vi "Main.vi"(7 "sweep rate, /min":dbl=0.2, 8 "sweep to:":dbl=-0.5, 9 "sweep":T3(radio)=enum."time_sweep") -> ()   [LabVIEW 2017] (continued)
                    n1197 = Build Array (concatenate)(w1474, w1473) -> (w1472:string[])
                    n1198 = Concatenate Strings(w1477, w1473, "\t") -> (w1476:string)
                  }
                }
                n1199 = property on="Figure_axis" class="Arr (strict)"("Value"=w1465) -> ()  [unwired: 2 in, 2 out]
                n1200 = property on="data_caption" class="Str"("Value"=w1467) -> ()  [unwired: 2 in, 2 out]
              }
              frame #14 {
                # "2182A 1 channel 1 measure (2182A_1_ch1)"
                n1201 = local read "2182A 1 ch1"() -> (w1484:bool)
                n1202 = property on="Figure_axis" class="Arr (strict)"() -> ("Value"=w1481:string[])  [unwired: 2 in, 2 out]
                n1203 = property on="data_caption" class="Str"() -> ("Value"=w1483:string)  [unwired: 2 in, 2 out]
                n1204 = case shown="False" w1484 {
                  tunnel: w1483 -> [w1486 w1492]
                  tunnel: [w1486 w1491] -> w1482
                  tunnel: w1481 -> [w1485 w1489]
                  tunnel: [w1485 w1487] -> w1480
                  frame False {
                    # "not measure 2182A 1 channel 1 (2182A_1_ch1)"
                  }
                  frame True {
                    w1488 = "2182A_1_ch1"
                    # "measure 2182A 1 channel 1 (2182A_1_ch1)"
                    n1205 = local read "2182A 1 addr"() -> (w1493:u8)
                    n1206 = Number To Decimal String(number=w1493) -> (decimal integer string=w1494:string)  [unwired: 1 in]
                    n1207 = GPIB Clear(3:w1494) -> ()  [unwired: 1 in, 2 out]
                    n1208 = Build Array (concatenate)(w1489, w1488) -> (w1487:string[])
                    n1209 = Concatenate Strings(w1492, w1488, "\t") -> (w1491:string)
                  }
                }
                n1210 = property on="Figure_axis" class="Arr (strict)"("Value"=w1480) -> ()  [unwired: 2 in, 2 out]
                n1211 = property on="data_caption" class="Str"("Value"=w1482) -> ()  [unwired: 2 in, 2 out]
              }
              frame #15 {
                # "2182A 1 channel 2 measure (2182A_1_ch2)"
                n1212 = local read "2182A 1 ch2"() -> (w1499:bool)
                n1213 = property on="Figure_axis" class="Arr (strict)"() -> ("Value"=w1496:string[])  [unwired: 2 in, 2 out]
                n1214 = property on="data_caption" class="Str"() -> ("Value"=w1498:string)  [unwired: 2 in, 2 out]
                n1215 = case shown="True" w1499 {
                  tunnel: w1498 -> [w1501 w1507]
                  tunnel: [w1501 w1506] -> w1497
                  tunnel: w1496 -> [w1500 w1504]
                  tunnel: [w1500 w1502] -> w1495
                  frame False {
                    # "not measure 2182A 1 channel 2 (2182A_1_ch2)"
                  }
                  frame True {
                    w1503 = "2182A_1_ch2"
                    # "measure 2182A 1 channel 2 (2182A_1_ch2)"
                    n1216 = local read "2182A 1 addr"() -> (w1508:u8)
                    n1217 = Number To Decimal String(number=w1508) -> (decimal integer string=w1509:string)  [unwired: 1 in]
                    n1218 = GPIB Clear(3:w1509) -> ()  [unwired: 1 in, 2 out]
                    n1219 = Build Array (concatenate)(w1504, w1503) -> (w1502:string[])
                    n1220 = Concatenate Strings(w1507, w1503, "\t") -> (w1506:string)
                  }
                }
                n1221 = property on="Figure_axis" class="Arr (strict)"("Value"=w1495) -> ()  [unwired: 2 in, 2 out]
                n1222 = property on="data_caption" class="Str"("Value"=w1497) -> ()  [unwired: 2 in, 2 out]
              }
              frame #16 {
                # "2182A 2 channel 1 measure (2182A_2_ch1)"
                n1223 = local read "2182A 2 ch1"() -> (w1514:bool)
                n1224 = property on="Figure_axis" class="Arr (strict)"() -> ("Value"=w1511:string[])  [unwired: 2 in, 2 out]
                n1225 = property on="data_caption" class="Str"() -> ("Value"=w1513:string)  [unwired: 2 in, 2 out]
                n1226 = case shown="True" w1514 {
                  tunnel: w1513 -> [w1516 w1522]
                  tunnel: [w1516 w1521] -> w1512
                  tunnel: w1511 -> [w1515 w1519]
                  tunnel: [w1515 w1517] -> w1510
                  frame False {
                    # "not measure 2182A 2 channel 1 (2182A_2_ch1)"
                  }
                  frame True {
                    w1518 = "2182A_2_ch1"
                    # "measure 2182A 2 channel 1 (2182A_2_ch1)"
                    n1227 = local read "2182A 2 addr"() -> (w1523:u8)
                    n1228 = Number To Decimal String(number=w1523) -> (decimal integer string=w1524:string)  [unwired: 1 in]
                    n1229 = GPIB Clear(3:w1524) -> ()  [unwired: 1 in, 2 out]
                    n1230 = Build Array (concatenate)(w1519, w1518) -> (w1517:string[])
                    n1231 = Concatenate Strings(w1522, w1518, "\t") -> (w1521:string)
                  }
                }
                n1232 = property on="Figure_axis" class="Arr (strict)"("Value"=w1510) -> ()  [unwired: 2 in, 2 out]
                n1233 = property on="data_caption" class="Str"("Value"=w1512) -> ()  [unwired: 2 in, 2 out]
              }
              frame #17 {
                # "2182A 2 channel 2 measure (2182A_2_ch2)"
                n1234 = local read "2182A 2 ch2"() -> (w1529:bool)
                n1235 = property on="Figure_axis" class="Arr (strict)"() -> ("Value"=w1526:string[])  [unwired: 2 in, 2 out]
                n1236 = property on="data_caption" class="Str"() -> ("Value"=w1528:string)  [unwired: 2 in, 2 out]
                n1237 = case shown="True" w1529 {
                  tunnel: w1528 -> [w1531 w1537]
                  tunnel: [w1531 w1536] -> w1527
                  tunnel: w1526 -> [w1530 w1534]
                  tunnel: [w1530 w1532] -> w1525
                  frame False {
                    # "not measure 2182A 2 channel 2 (2182A_2_ch2)"
                  }
                  frame True {
                    w1533 = "2182A_2_ch2"
                    # "measure 2182A 2 channel 2 (2182A_2_ch2)"
                    n1238 = local read "2182A 2 addr"() -> (w1538:u8)
                    n1239 = Number To Decimal String(number=w1538) -> (decimal integer string=w1539:string)  [unwired: 1 in]
                    n1240 = GPIB Clear(3:w1539) -> ()  [unwired: 1 in, 2 out]
                    n1241 = Build Array (concatenate)(w1534, w1533) -> (w1532:string[])
                    n1242 = Concatenate Strings(w1537, w1533, "\t") -> (w1536:string)
                  }
                }
                n1243 = property on="Figure_axis" class="Arr (strict)"("Value"=w1525) -> ()  [unwired: 2 in, 2 out]
                n1244 = property on="data_caption" class="Str"("Value"=w1527) -> ()  [unwired: 2 in, 2 out]
              }
              frame #18 {
                # "2182A 3 channel 1 measure (2182A_3_ch1)"
                n1245 = local read "2182A 3 ch1"() -> (w1544:bool)
                n1246 = property on="Figure_axis" class="Arr (strict)"() -> ("Value"=w1541:string[])  [unwired: 2 in, 2 out]
                n1247 = property on="data_caption" class="Str"() -> ("Value"=w1543:string)  [unwired: 2 in, 2 out]
                n1248 = case shown="True" w1544 {
                  tunnel: w1543 -> [w1546 w1552]
                  tunnel: [w1546 w1551] -> w1542
                  tunnel: w1541 -> [w1545 w1549]
                  tunnel: [w1545 w1547] -> w1540
                  frame False {
                    # "not measure 2182A 3 channel 1 (2182A_3_ch1)"
                  }
                  frame True {
                    w1548 = "2182A_3_ch1"
                    # "measure 2182A 3 channel 1 (2182A_3_ch1)"
                    n1249 = local read "2182A 3 addr"() -> (w1553:u8)
                    n1250 = Number To Decimal String(number=w1553) -> (decimal integer string=w1554:string)  [unwired: 1 in]
                    n1251 = GPIB Clear(3:w1554) -> ()  [unwired: 1 in, 2 out]
                    n1252 = Build Array (concatenate)(w1549, w1548) -> (w1547:string[])
                    n1253 = Concatenate Strings(w1552, w1548, "\t") -> (w1551:string)
                  }
                }
                n1254 = property on="Figure_axis" class="Arr (strict)"("Value"=w1540) -> ()  [unwired: 2 in, 2 out]
                n1255 = property on="data_caption" class="Str"("Value"=w1542) -> ()  [unwired: 2 in, 2 out]
              }
              frame #19 {
                # "2182A 3 channel 2 measure (2182A_3_ch2)"
                n1256 = local read "2182A 3 ch2"() -> (w1559:bool)
                n1257 = property on="Figure_axis" class="Arr (strict)"() -> ("Value"=w1556:string[])  [unwired: 2 in, 2 out]
                n1258 = property on="data_caption" class="Str"() -> ("Value"=w1558:string)  [unwired: 2 in, 2 out]
                n1259 = case shown="False" w1559 {
                  tunnel: w1558 -> [w1561 w1567]
                  tunnel: [w1561 w1566] -> w1557
                  tunnel: w1556 -> [w1560 w1564]
                  tunnel: [w1560 w1562] -> w1555
                  frame False {
                    # "not measure 2182A 3 channel 2 (2182A_3_ch2)"
                  }
                  frame True {
                    w1563 = "2182A_3_ch2"
                    # "measure 2182A 3 channel 2 (2182A_3_ch2)"
                    n1260 = local read "2182A 3 addr"() -> (w1568:u8)
                    n1261 = Number To Decimal String(number=w1568) -> (decimal integer string=w1569:string)  [unwired: 1 in]
                    n1262 = GPIB Clear(3:w1569) -> ()  [unwired: 1 in, 2 out]
                    n1263 = Build Array (concatenate)(w1564, w1563) -> (w1562:string[])
                    n1264 = Concatenate Strings(w1567, w1563, "\t") -> (w1566:string)
                  }
                }
                n1265 = property on="Figure_axis" class="Arr (strict)"("Value"=w1555) -> ()  [unwired: 2 in, 2 out]
                n1266 = property on="data_caption" class="Str"("Value"=w1557) -> ()  [unwired: 2 in, 2 out]
              }
              frame #20 {
                # "2182A 4 channel 1 measure (2182A_4_ch1)"
                n1267 = local read "2182A 4 ch1"() -> (w1574:bool)
                n1268 = property on="Figure_axis" class="Arr (strict)"() -> ("Value"=w1571:string[])  [unwired: 2 in, 2 out]
                n1269 = property on="data_caption" class="Str"() -> ("Value"=w1573:string)  [unwired: 2 in, 2 out]
                n1270 = case shown="True" w1574 {
                  tunnel: w1573 -> [w1576 w1582]
                  tunnel: [w1576 w1581] -> w1572
                  tunnel: w1571 -> [w1575 w1579]
                  tunnel: [w1575 w1577] -> w1570
                  frame False {
                    # "not measure 2182A 4 channel 1 (2182A_4_ch1)"
                  }
                  frame True {
                    w1578 = "2182A_4_ch1"
                    # "measure 2182A 4 channel 1 (2182A_4_ch1)"
                    n1271 = local read "2182A 4 addr"() -> (w1583:u8)
                    n1272 = Number To Decimal String(number=w1583) -> (decimal integer string=w1584:string)  [unwired: 1 in]
                    n1273 = GPIB Clear(3:w1584) -> ()  [unwired: 1 in, 2 out]
                    n1274 = Build Array (concatenate)(w1579, w1578) -> (w1577:string[])
                    n1275 = Concatenate Strings(w1582, w1578, "\t") -> (w1581:string)
                  }
                }
                n1276 = property on="Figure_axis" class="Arr (strict)"("Value"=w1570) -> ()  [unwired: 2 in, 2 out]
                n1277 = property on="data_caption" class="Str"("Value"=w1572) -> ()  [unwired: 2 in, 2 out]
              }
              frame #21 {
                # "2182A 4 channel 2 measure (2182A_4_ch2)"
                n1278 = local read "2182A 4 ch2"() -> (w1589:bool)
                n1279 = property on="Figure_axis" class="Arr (strict)"() -> ("Value"=w1586:string[])  [unwired: 2 in, 2 out]
                n1280 = property on="data_caption" class="Str"() -> ("Value"=w1588:string)  [unwired: 2 in, 2 out]
                n1281 = case shown="True" w1589 {
                  tunnel: w1588 -> [w1591 w1597]
                  tunnel: [w1591 w1596] -> w1587
                  tunnel: w1586 -> [w1590 w1594]
                  tunnel: [w1590 w1592] -> w1585
                  frame False {
                    # "not measure 2182A 4 channel 2 (2182A_4_ch2)"
                  }
                  frame True {
                    w1593 = "2182A_4_ch2"
                    # "measure 2182A 4 channel 2 (2182A_4_ch2)"
                    n1282 = local read "2182A 4 addr"() -> (w1598:u8)
                    n1283 = Number To Decimal String(number=w1598) -> (decimal integer string=w1599:string)  [unwired: 1 in]
                    n1284 = GPIB Clear(3:w1599) -> ()  [unwired: 1 in, 2 out]
                    n1285 = Build Array (concatenate)(w1594, w1593) -> (w1592:string[])
                    n1286 = Concatenate Strings(w1597, w1593, "\t") -> (w1596:string)
                  }
                }
                n1287 = property on="Figure_axis" class="Arr (strict)"("Value"=w1585) -> ()  [unwired: 2 in, 2 out]
                n1288 = property on="data_caption" class="Str"("Value"=w1587) -> ()  [unwired: 2 in, 2 out]
              }
              frame #22 {
                # "2636A smua measure voltage (2636A_smua_v)"
                n1289 = local read "2636A smua meas v"() -> (w1604:bool)
                n1290 = property on="Figure_axis" class="Arr (strict)"() -> ("Value"=w1601:string[])  [unwired: 2 in, 2 out]
                n1291 = property on="data_caption" class="Str"() -> ("Value"=w1603:string)  [unwired: 2 in, 2 out]
                n1292 = case shown="True" w1604 {
                  tunnel: w1603 -> [w1606 w1617]
                  tunnel: [w1606 w1616] -> w1602
                  tunnel: w1601 -> [w1605 w1614]
                  tunnel: [w1605 w1612] -> w1600
                  frame False {
                    # "not measure voltage on 2636A smua (2636A_smua_v)"
                  }
                  frame True {
                    w1613 = "2636A_smua_v"
                    # "measure voltage on 2636A smua (2636A_smua_v)"
                    n1293 = local read "2336A addr"() -> (w1608:refnum<visa-resource-name>)
                    n1294 = VISA Open(VISA resource name=w1608) -> (VISA resource name=w1607:refnum<visa-resource-name>, error out=w1609:errorcluster)  [unwired: 4 in]
                    n1295 = VISA Clear(VISA resource name=w1607, error in (no error)=w1609) -> (VISA resource name out=w1611:refnum<visa-resource-name>)  [unwired: 1 out]
                    n1296 = property class="Instr"(reference=w1611, "General Settings:Timeout Value"=u32 10000) -> ()  [unwired: 1 in, 2 out]
                    n1297 = Build Array (concatenate)(w1614, w1613) -> (w1612:string[])
                    n1298 = Concatenate Strings(w1617, w1613, "\t") -> (w1616:string)
                  }
                }
                n1299 = property on="Figure_axis" class="Arr (strict)"("Value"=w1600) -> ()  [unwired: 2 in, 2 out]
                n1300 = property on="data_caption" class="Str"("Value"=w1602) -> ()  [unwired: 2 in, 2 out]
              }
              frame #23 {
                # "2636A smua measure current (2636A_smua_i)"
                n1301 = local read "2636A smua meas i"() -> (w1622:bool)
                n1302 = property on="Figure_axis" class="Arr (strict)"() -> ("Value"=w1619:string[])  [unwired: 2 in, 2 out]
                n1303 = property on="data_caption" class="Str"() -> ("Value"=w1621:string)  [unwired: 2 in, 2 out]
                n1304 = case shown="True" w1622 {
                  tunnel: w1621 -> [w1624 w1635]
                  tunnel: [w1624 w1634] -> w1620
                  tunnel: w1619 -> [w1623 w1632]
                  tunnel: [w1623 w1630] -> w1618
                  frame False {
                    # "not measure current on 2636A smua (2636A_smua_i)"
                  }
                  frame True {
                    w1631 = "2636A_smua_i"
                    # "measure current on 2636A smua (2636A_smua_i)"
                    n1305 = local read "2336A addr"() -> (w1627:refnum<visa-resource-name>)
                    n1306 = VISA Open(VISA resource name=w1627) -> (VISA resource name=w1626:refnum<visa-resource-name>, error out=w1625:errorcluster)  [unwired: 4 in]
                    n1307 = VISA Clear(VISA resource name=w1626, error in (no error)=w1625) -> (VISA resource name out=w1628:refnum<visa-resource-name>)  [unwired: 1 out]
                    n1308 = Build Array (concatenate)(w1632, w1631) -> (w1630:string[])
                    n1309 = property class="Instr"(reference=w1628, "General Settings:Timeout Value"=u32 10000) -> ()  [unwired: 1 in, 2 out]
                    n1310 = Concatenate Strings(w1635, w1631, "\t") -> (w1634:string)
                  }
                }
                n1311 = property on="Figure_axis" class="Arr (strict)"("Value"=w1618) -> ()  [unwired: 2 in, 2 out]
                n1312 = property on="data_caption" class="Str"("Value"=w1620) -> ()  [unwired: 2 in, 2 out]
              }
              frame #24 {
                # "2636A smub measure voltage (2636A_smub_v)"
                n1313 = local read "2636A smub meas v"() -> (w1640:bool)
                n1314 = property on="Figure_axis" class="Arr (strict)"() -> ("Value"=w1637:string[])  [unwired: 2 in, 2 out]
                n1315 = property on="data_caption" class="Str"() -> ("Value"=w1639:string)  [unwired: 2 in, 2 out]
                n1316 = case shown="True" w1640 {
                  tunnel: w1639 -> [w1642 w1653]
                  tunnel: [w1642 w1652] -> w1638
                  tunnel: w1637 -> [w1641 w1650]
                  tunnel: [w1641 w1648] -> w1636
                  frame False {
                    # "not measure voltage on 2636A smub (2636A_smub_v)"
                  }
                  frame True {
                    w1649 = "2636A_smub_v"
                    # "measure voltage on 2636A smub (2636A_smub_v)"
                    n1317 = local read "2336A addr"() -> (w1644:refnum<visa-resource-name>)
                    n1318 = VISA Open(VISA resource name=w1644) -> (VISA resource name=w1643:refnum<visa-resource-name>, error out=w1645:errorcluster)  [unwired: 4 in]
                    n1319 = VISA Clear(VISA resource name=w1643, error in (no error)=w1645) -> (VISA resource name out=w1646:refnum<visa-resource-name>)  [unwired: 1 out]
                    n1320 = Build Array (concatenate)(w1650, w1649) -> (w1648:string[])
                    n1321 = property class="Instr"(reference=w1646, "General Settings:Timeout Value"=u32 10000) -> ()  [unwired: 1 in, 2 out]
                    n1322 = Concatenate Strings(w1653, w1649, "\t") -> (w1652:string)
                  }
                }
                n1323 = property on="Figure_axis" class="Arr (strict)"("Value"=w1636) -> ()  [unwired: 2 in, 2 out]
                n1324 = property on="data_caption" class="Str"("Value"=w1638) -> ()  [unwired: 2 in, 2 out]
              }
              frame #25 {
                # "2636A smub measure current (2636A_smub_i)"
                n1325 = local read "2636A smub meas i"() -> (w1658:bool)
                n1326 = property on="Figure_axis" class="Arr (strict)"() -> ("Value"=w1655:string[])  [unwired: 2 in, 2 out]
                n1327 = property on="data_caption" class="Str"() -> ("Value"=w1657:string)  [unwired: 2 in, 2 out]
                n1328 = case shown="True" w1658 {
                  tunnel: w1657 -> [w1660 w1671]
                  tunnel: [w1660 w1670] -> w1656
                  tunnel: w1655 -> [w1659 w1668]
                  tunnel: [w1659 w1666] -> w1654
                  frame False {
                    # "not measure current on 2636A smub (2636A_smub_i)"
                  }
                  frame True {
                    w1667 = "2636A_smub_i"
                    # "measure current on 2636A smub (2636A_smub_i)"
                    n1329 = local read "2336A addr"() -> (w1661:refnum<visa-resource-name>)
                    n1330 = VISA Open(VISA resource name=w1661) -> (VISA resource name=w1662:refnum<visa-resource-name>, error out=w1663:errorcluster)  [unwired: 4 in]
                    n1331 = VISA Clear(VISA resource name=w1662, error in (no error)=w1663) -> (VISA resource name out=w1664:refnum<visa-resource-name>)  [unwired: 1 out]
                    n1332 = Build Array (concatenate)(w1668, w1667) -> (w1666:string[])
                    n1333 = property class="Instr"(reference=w1664, "General Settings:Timeout Value"=u32 10000) -> ()  [unwired: 1 in, 2 out]
                    n1334 = Concatenate Strings(w1671, w1667, "\t") -> (w1670:string)
                  }
                }
                n1335 = property on="Figure_axis" class="Arr (strict)"("Value"=w1654) -> ()  [unwired: 2 in, 2 out]
                n1336 = property on="data_caption" class="Str"("Value"=w1656) -> ()  [unwired: 2 in, 2 out]
              }
              frame #26 {
                # "measure time"
                n1337 = local read "measure time"() -> (w1676:bool)
                n1338 = property on="Figure_axis" class="Arr (strict)"() -> ("Value"=w1673:string[])  [unwired: 2 in, 2 out]
                n1339 = property on="data_caption" class="Str"() -> ("Value"=w1675:string)  [unwired: 2 in, 2 out]
                n1340 = case shown="True" w1676 {
                  tunnel: w1675 -> [w1678 w1684]
                  tunnel: [w1678 w1683] -> w1674
                  tunnel: w1673 -> [w1677 w1681]
                  tunnel: [w1677 w1679] -> w1672
                  frame False {
                    # "not measuring time"
                  }
                  frame True {
                    w1680 = "time"
                    # "measuring time"
                    n1341 = Build Array (concatenate)(w1681, w1680) -> (w1679:string[])
                    n1342 = Concatenate Strings(w1684, w1680, "\t") -> (w1683:string)
                  }
                }
                n1343 = property on="Figure_axis" class="Arr (strict)"("Value"=w1672) -> ()  [unwired: 2 in, 2 out]
                n1344 = property on="data_caption" class="Str"("Value"=w1674) -> ()  [unwired: 2 in, 2 out]
              }
              frame #27 {
                # "Measure magnetic field on IPS120-0"
                n1345 = local read "iPS_MagnetField"() -> (w1689:bool)
                n1346 = property on="Figure_axis" class="Arr (strict)"() -> ("Value"=w1686:string[])  [unwired: 2 in, 2 out]
                n1347 = property on="data_caption" class="Str"() -> ("Value"=w1688:string)  [unwired: 2 in, 2 out]
                n1348 = case shown="True" w1689 {
                  tunnel: w1688 -> [w1691 w1699]
                  tunnel: [w1691 w1698] -> w1687
                  tunnel: w1686 -> [w1690 w1696]
                  tunnel: [w1690 w1694] -> w1685
                  frame False {
                    # "do not Measure magnetic field on IPS120-0"
                  }
                  frame True {
                    w1695 = "iPS_MagntField"
                    n1349 = local read "IPS120-0 addr_sweep"() -> (w1693:u8)
                    n1350 = Number To Decimal String(number=w1693) -> (decimal integer string=w1692:string)  [unwired: 1 in]
                    n1351 = GPIB Clear(3:w1692) -> ()  [unwired: 1 in, 2 out]
                    n1352 = Build Array (concatenate)(w1696, w1695) -> (w1694:string[])
                    n1353 = Concatenate Strings(w1699, w1695, "\t") -> (w1698:string)
                  }
                }
                n1354 = property on="Figure_axis" class="Arr (strict)"("Value"=w1685) -> ()  [unwired: 2 in, 2 out]
                n1355 = property on="data_caption" class="Str"("Value"=w1687) -> ()  [unwired: 2 in, 2 out]
              }
              frame #28 {
                # "iTC sample Temp"
                n1356 = property on="iTC_Sample_T" class="Bool (strict)"() -> ("Value"=w1700:bool)  [unwired: 2 in, 2 out]
                n1357 = property on="Figure_axis" class="Arr (strict)"() -> ("Value"=w1702:string[])  [unwired: 2 in, 2 out]
                n1358 = property on="data_caption" class="Str"() -> ("Value"=w1704:string)  [unwired: 2 in, 2 out]
                n1359 = case shown="True" w1700 {
                  tunnel: w1704 -> [w1706 w1714]
                  tunnel: [w1706 w1713] -> w1703
                  tunnel: w1702 -> [w1705 w1711]
                  tunnel: [w1705 w1709] -> w1701
                  frame False {
                    # "not measure 2461 voltage (2461_meas_v)"
                  }
                  frame True {
                    w1710 = "iTC_Sample_T"
                    n1360 = local read "ITC503S addr_step"() -> (w1708:u8)
                    n1361 = Number To Decimal String(number=w1708) -> (decimal integer string=w1707:string)  [unwired: 1 in]
                    n1362 = GPIB Clear(3:w1707) -> ()  [unwired: 1 in, 2 out]
                    n1363 = Build Array (concatenate)(w1711, w1710) -> (w1709:string[])
                    n1364 = Concatenate Strings(w1714, w1710, "\t") -> (w1713:string)
                  }
                }
                n1365 = property on="Figure_axis" class="Arr (strict)"("Value"=w1701) -> ()  [unwired: 2 in, 2 out]
                n1366 = property on="data_caption" class="Str"("Value"=w1703) -> ()  [unwired: 2 in, 2 out]
              }
              frame #29 {
                # "iTC CH_A Temp"
                n1367 = property on="CH_A" class="Bool (strict)"() -> ("Value"=w1715:bool)  [unwired: 2 in, 2 out]
                n1368 = property on="Figure_axis" class="Arr (strict)"() -> ("Value"=w1717:string[])  [unwired: 2 in, 2 out]
                n1369 = property on="data_caption" class="Str"() -> ("Value"=w1719:string)  [unwired: 2 in, 2 out]
                n1370 = case shown="True" w1715 {
                  tunnel: w1719 -> [w1721 w1727]
                  tunnel: [w1721 w1726] -> w1718
                  tunnel: w1717 -> [w1720 w1724]
                  tunnel: [w1720 w1722] -> w1716
                  frame False {
                    # "not measure 2461 voltage (2461_meas_v)"
                  }
                  frame True {
                    w1723 = "iTC_CH_A"
                    n1371 = Build Array (concatenate)(w1724, w1723) -> (w1722:string[])
                    n1372 = Concatenate Strings(w1727, w1723, "\t") -> (w1726:string)
                  }
                }
                n1373 = property on="Figure_axis" class="Arr (strict)"("Value"=w1716) -> ()  [unwired: 2 in, 2 out]
                n1374 = property on="data_caption" class="Str"("Value"=w1718) -> ()  [unwired: 2 in, 2 out]
              }
              frame #30 {
                # "iTC sample Temp"
                n1375 = property on="CH_B" class="Bool (strict)"() -> ("Value"=w1728:bool)  [unwired: 2 in, 2 out]
                n1376 = property on="Figure_axis" class="Arr (strict)"() -> ("Value"=w1730:string[])  [unwired: 2 in, 2 out]
                n1377 = property on="data_caption" class="Str"() -> ("Value"=w1732:string)  [unwired: 2 in, 2 out]
                n1378 = case shown="True" w1728 {
                  tunnel: w1732 -> [w1734 w1740]
                  tunnel: [w1734 w1739] -> w1731
                  tunnel: w1730 -> [w1733 w1737]
                  tunnel: [w1733 w1735] -> w1729
                  frame False {
                    # "not measure 2461 voltage (2461_meas_v)"
                  }
                  frame True {
                    w1736 = "iTC_CH_B"
                    n1379 = Build Array (concatenate)(w1737, w1736) -> (w1735:string[])
                    n1380 = Concatenate Strings(w1740, w1736, "\t") -> (w1739:string)
                  }
                }
                n1381 = property on="Figure_axis" class="Arr (strict)"("Value"=w1729) -> ()  [unwired: 2 in, 2 out]
                n1382 = property on="data_caption" class="Str"("Value"=w1731) -> ()  [unwired: 2 in, 2 out]
              }
              frame #31 {
                # "iTC sample Temp"
                n1383 = property on="Linetrace or Mapping?" class="Bool (strict)"() -> ("Value"=w1741:bool)  [unwired: 2 in, 2 out]
                n1384 = property on="Figure_axis" class="Arr (strict)"() -> ("Value"=w1743:string[])  [unwired: 2 in, 2 out]
                n1385 = property on="data_caption" class="Str"() -> ("Value"=w1745:string)  [unwired: 2 in, 2 out]
                n1386 = case shown="True" w1741 {
                  tunnel: w1745 -> [w1747 w1753]
                  tunnel: [w1747 w1752] -> w1744
                  tunnel: w1743 -> [w1746 w1750]
                  tunnel: [w1746 w1748] -> w1742
                  frame False {
                    # "not measure 2461 voltage (2461_meas_v)"
                  }
                  frame True {
                    w1749 = "Step_Value"
                    n1387 = Build Array (concatenate)(w1750, w1749) -> (w1748:string[])
                    n1388 = Concatenate Strings(w1753, w1749, "\t") -> (w1752:string)
                  }
                }
                n1389 = property on="Figure_axis" class="Arr (strict)"("Value"=w1742) -> ()  [unwired: 2 in, 2 out]
                n1390 = property on="data_caption" class="Str"("Value"=w1744) -> ()  [unwired: 2 in, 2 out]
              }
            }
          }
          frame #2 {
            # "1 = 2400 1\n2 = 2400 2\n3 = 2400 3\n4 = 2636a smua\n5 = 2636a smub\n6 = do not sweep, just time\n7 = Teslatron_iPS_Field\n8 = Teslatron_iTC_Sample T"
            n1391 = property on="sweep" class="RadioBtnsControl (strict)"() -> ("Value"=w1754:T3)  [unwired: 2 in, 2 out]
            n1392 = case "reads current value from instrument which will be sweeping" shown="\"2636a_smub\"" w1754 {
              tunnel: [w1756 w1766 w1775 w1784 w1788 0.0 ("Measuremet") w1794 w1795] -> w1755
              frame "2400_1", Default {
                # "reads the voltage on 2400 1"
                n1393 = local read "2400 1 addr"() -> (w1760:u8)
                n1394 = Number To Decimal String(number=w1760) -> (decimal integer string=w1761:string)  [unwired: 1 in]
                n1395 = GPIB Write(0:w1761, 1:":READ?") -> (6:w1757:errorcluster)  [unwired: 3 in, 1 out]
                n1396 = GPIB Read(0:w1761, 1:3200, 3:w1757) -> (5:w1763:string)  [unwired: 2 in, 2 out]
                n1397 = String Subset(string=w1763, length (rest)=13) -> (substring=w1764:string)  [unwired: 1 in]
                n1398 = Fract/Exp String To Number(string=w1764) -> (number=w1756:dbl)  [unwired: 3 in, 1 out]
              }
              frame "2400_2" {
                # "reads the current on 2400 2"
                n1399 = local read "2400 2 addr"() -> (w1770:u8)
                n1400 = Number To Decimal String(number=w1770) -> (decimal integer string=w1771:string)  [unwired: 1 in]
                n1401 = GPIB Write(0:w1771, 1:":READ?") -> (6:w1767:errorcluster)  [unwired: 3 in, 1 out]
                n1402 = GPIB Read(0:w1771, 1:3200, 3:w1767) -> (5:w1773:string)  [unwired: 2 in, 2 out]
                n1403 = String Subset(string=w1773, offset (0)=14, length (rest)=13) -> (substring=w1774:string)
                n1404 = Fract/Exp String To Number(string=w1774) -> (number=w1766:dbl)  [unwired: 3 in, 1 out]
              }
              frame "2400_3" {
                # "reads the voltage on 2400 3"
                n1405 = local read "2400 3 addr"() -> (w1779:u8)
                n1406 = Number To Decimal String(number=w1779) -> (decimal integer string=w1780:string)  [unwired: 1 in]
                n1407 = GPIB Write(0:w1780, 1:":READ?") -> (6:w1776:errorcluster)  [unwired: 3 in, 1 out]
                n1408 = GPIB Read(0:w1780, 1:3200, 3:w1776) -> (5:w1782:string)  [unwired: 2 in, 2 out]
                n1409 = String Subset(string=w1782, length (rest)=13) -> (substring=w1783:string)  [unwired: 1 in]
                n1410 = Fract/Exp String To Number(string=w1783) -> (number=w1775:dbl)  [unwired: 3 in, 1 out]
              }
              frame "2636a_smua" {
                # "reads the voltage on 2636a smua"
                n1411 = local read "2336A addr"() -> (w1787:refnum<visa-resource-name>)
                n1412 = call "SinglePointMeasurement.vi"("Measure"=Measure."Voltage", "Channel"=Channel."a", "VISA resource name 2"=w1787) -> ("Measuremet"=w1784:dbl)  [unwired: 3 in, 4 out]
              }
              frame "2636a_smub" {
                # "reads the voltage on 2636a smub"
                n1413 = local read "2336A addr"() -> (w1791:refnum<visa-resource-name>)
                n1414 = call "SinglePointMeasurement.vi"("Measure"=Measure."Voltage", "Channel"=Channel."b", "VISA resource name 2"=w1791) -> ("Measuremet"=w1788:dbl)  [unwired: 3 in, 4 out]
              }
              frame "time_sweep" {
              }
              frame "iPS" {
                # "Measure magnetic field on IPS120-0"
                n1415 = call "iPSread.vi"("iPSreadCtrl"=iPSreadCtrl."OutputField") -> ("number"=w1794:dbl)  [unwired: 7 in, 3 out]
              }
              frame "iTC" {
                n1416 = call "iTCread.vi"("iTCreadCtrl"=iTCreadCtrl."Sample Temp") -> ("number"=w1795:dbl)  [unwired: 6 in, 3 out]
              }
            }
          }
          frame #3 {
            n1417 = property on="Linetrace or Mapping?" class="Bool (strict)"() -> ("Value"=w1797:bool)  [unwired: 2 in, 2 out]
            n1418 = case shown="True" w1797 {
              frame False {
                # "Reserve a name for new linetrace data file:"
                n1419 = property on="Data Folder" class="Path"() -> ("Value"=w1805:path)  [unwired: 2 in, 2 out]
                n1420 = call "AutoNamerDatExtraArtem.vi"("SweepType"="linetraces", "Custom User Path"=w1805) -> ("String"=w1803:string, "Path"=w1804:path)  [unwired: 2 in]
                n1421 = Path To String(path=w1804) -> (string=w1802:string)
                n1422 = Concatenate Strings(w1802, "\\", w1803) -> (w1801:string)
                n1423 = String To Path(string=w1801) -> (path=w1800:path)
                n1424 = local write "Data file:"(w1800) -> ()
              }
              frame True {
                n1425 = property on="Sweep Direction" class="Str"() -> ("Value"=w1806:string)  [unwired: 2 in, 2 out]
                n1426 = case shown="\"Sweep Down\"" w1806 {
                  frame "Sweep Up" {
                    n1427 = property on="UpNameString" class="Str"() -> ("Value"=w1808:string)  [unwired: 2 in, 2 out]
                    n1428 = String To Path(string=w1808) -> (path=w1807:path)
                    n1429 = local write "Data file:"(w1807) -> ()
                  }
                  frame "Sweep Down" {
                    n1430 = property on="DownNameString" class="Str"() -> ("Value"=w1809:string)  [unwired: 2 in, 2 out]
                    n1431 = String To Path(string=w1809) -> (path=w1810:path)
                    n1432 = local write "Data file:"(w1810) -> ()
                  }
                  frame "Ramp Down", Default {
                  }
                }
              }
            }
          }
          frame #4 {
            # "add \"formula\" string to the axis rings"
            n1433 = property on="Figure_axis" class="Arr (strict)"() -> ("Value"=w1813:string[])  [unwired: 2 in, 2 out]
            n1434 = Build Array (concatenate)(w1813, "formula") -> (w1811:string[])
            n1435 = property on="Figure_axis" class="Arr (strict)"("Value"=w1811) -> ()  [unwired: 2 in, 2 out]
          }
          frame #5 {
            # "passes array to ring"
            n1436 = property on="Linetrace or Mapping?" class="Bool (strict)"() -> ("Value"=w1814:bool)  [unwired: 2 in, 2 out]
            n1437 = case shown="True" w1814 {
              frame False {
                # "records the fist line into the data file"
                n1438 = property on="data_caption" class="Str"() -> ("Value"=w1818:string)  [unwired: 2 in, 2 out]
                n1439 = local read "Data file:"() -> (w1819:path)
                n1440 = Concatenate Strings(w1818, "\r") -> (w1820:string)
                n1441 = Write to Text File(file (use dialog)=w1819, text=w1820) -> ()  [unwired: 2 in, 3 out]
              }
              frame True {
                # "records the fist line into the both upa nd down data file\nwhen table index=0"
                n1442 = property on="Table Index" class="DigNum (strict)"() -> ("Value"=w1822:dbl)  [unwired: 2 in, 2 out]
                n1443 = Equal To 0?(x=w1822) -> (x = 0?=w1821:bool)
                n1444 = case shown="True" w1821 {
                  frame False {
                  }
                  frame True {
                    n1445 = property on="data_caption" class="Str"() -> ("Value"=w1826:string)  [unwired: 2 in, 2 out]
                    n1446 = local read "Data file:"() -> (w1823:path)
                    n1447 = Concatenate Strings(w1826, "\r") -> (w1825:string)
                    n1448 = Write to Text File(file (use dialog)=w1823, text=w1825) -> ()  [unwired: 2 in, 3 out]
                  }
                }
              }
            }
            n1449 = property on="Figure_axis" class="Arr (strict)"() -> ("Value"=w1816:string[])  [unwired: 2 in, 2 out]
            n1450 = property on="Xaxis" class="Ring (strict)"("Strings []"=w1816) -> ()  [unwired: 2 in, 2 out]
            n1451 = property on="Stop Sweep" class="Bool"("DisabledEnum"=T5."Enabled" ("Disabled")) -> ()  [unwired: 2 in, 2 out]
            n1452 = property on="Yright" class="Ring (strict)"("Strings []"=w1816) -> ()  [unwired: 2 in, 2 out]
            n1453 = property on="Yaxis" class="Ring (strict)"("Strings []"=w1816) -> ()  [unwired: 2 in, 2 out]
          }
        }
        n1454 = while {
          shift-right: [w1877] -> _
          shift-left: w1212 -> [w1878]
          shift-right: [w1875] -> w1211
          shift-left: w1209 -> [w1874]
          tunnel: w1213 -> [w1872]
          stop <- w1864 stop-if-true
          # "initial value"
          # "Measure the selected channels"
          # "data array"
          # "this loop stops when target value is reached"
          # "error cluster to determine data flow"
          n1455 = stacked-sequence {
            tunnel: [_ _ w1894 _ _ _] -> w1865
            tunnel: [_ _ w1893 _ _ _] -> w1876
            tunnel: w1874 -> [_ _ w1888 _ _ _]
            tunnel: [w1884 _ _ _ _ _] -> w1873
            tunnel: w1872 -> [_ _ _ w1909 _ _]
            tunnel: [_ _ w1888 _ _ _] -> w1868
            tunnel: [_ _ _ _ _ w2369] -> w1863
            frame #0 {
              # "time is measured at the beginning\nand at the end of the cycle to\ncalculate delay time required to\nkeep set sweep rate"
              n1456 = flat-sequence {
                tunnel: [w1886] -> w1884
                frame #0 {
                  n1457 = property on="time delay, ms" class="DigNum (strict)"() -> ("Value"=w1885:dbl)  [unwired: 2 in, 2 out]
                  n1458 = Wait (ms)(milliseconds to wait=w1885) -> ()  [unwired: 1 out]
                }
                frame #1 {
                  n1459 = Tick Count (ms)() -> (millisecond timer value=w1886:u32)
                }
              }
            }
            frame #1 {
              w1887 = dbl[] []  # Empty array for data
              # "clear data array before each measurement cycle"
              n1460 = property on="data" class="Arr (strict)"("Value"=w1887) -> ()  [unwired: 2 in, 2 out]
            }
            frame #2 {
              # "add next sweep value to the data array"
              n1461 = property on="data" class="Arr (strict)"() -> ("Value"=w1892:dbl[])  [unwired: 2 in, 2 out]
              n1462 = case shown="False" FALSE {
                tunnel: [w1895 w1905] -> w1894
                tunnel: [w1896 w1904] -> w1893
                tunnel: w1888 -> [_ w1902]
                tunnel: [w1896 w1902] -> w1890
                frame True {
                  # "sweeping magnetic field of Hulk"
                  n1463 = stacked-sequence {
                    tunnel: [_ w1898 _] -> w1896
                    tunnel: [_ _ w1900] -> w1895
                    frame #0 {
                      n1464 = local read "Hulk_SMS_addr"() -> (w1897:refnum<visa-resource-name>)
                      n1465 = VISA Clear(VISA resource name=w1897) -> ()  [unwired: 1 in, 2 out]
                    }
                    frame #1 {
                      # "acquires current output value"
                      n1466 = local read "Hulk_SMS_addr"() -> (w1899:refnum<visa-resource-name>)
                      n1467 = call "SMS_GET_OUTPUT.vi"("Hulk_SMS_addr"=w1899) -> ("Numeric"=w1898:dbl)  [unwired: 1 in, 2 out]
                    }
                    frame #2 {
                      # "checks, wheter ramp was finished"
                      n1468 = local read "Hulk_SMS_addr"() -> (w1901:refnum<visa-resource-name>)
                      n1469 = call "SMS_RAMP_STATUS.vi"("Hulk_SMS_addr"=w1901) -> ("selection"=w1900:bool)  [unwired: 1 in, 2 out]
                    }
                  }
                }
                frame False {
                  # "calculate next value"
                  n1470 = call "CalculateNextValue.vi"("Target a 2"="sweep to:", "Channel a source value"=w1902, "Ch a sweep rate units/min"="sweep rate, /min", "time between points, sec"="time/point, sec", "Source a"=Source."Voltage") -> ("Target a"=w1904:dbl, "Boolean"=w1905:bool)
                }
              }
              n1471 = Build Array (concatenate)(w1892, w1890) -> (w1891:dbl[])
              n1472 = property on="data" class="Arr (strict)"("Value"=w1891) -> ()  [unwired: 2 in, 2 out]
            }
            frame #3 {
              n1473 = stacked-sequence "measurement sequence" {
                tunnel: w1909 -> [_ _ _ _ _ _ _ _ _ _ _ _ _ _ _ _ _ _ _ _ _ _ _ _ _ _ w2283 _ _ _ _ _]
                frame #0 {
                  # "check if in-phase\nsignal on lock-in 1 \nis to be measured"
                  n1474 = property on="data" class="Arr (strict)"() -> ("Value"=w1911:dbl[])  [unwired: 2 in, 2 out]
                  n1475 = local read "SR830 1 ip"() -> (w1910:bool)
                  n1476 = case shown="True" w1910 {
                    tunnel: w1911 -> [w1913 w1922]
                    tunnel: [w1913 w1921] -> w1912
                    frame False {
                      # "we are not measuring in phase signal on lock-in 1 (SR830_1_ip)"
                    }
                    frame True {
                      # "we are  measuring lock-in 1, in phase (SR830_1_ip)"
                      n1477 = local read "SR830 1 addr"() -> (w1915:u8)
                      n1478 = Number To Decimal String(number=w1915) -> (decimal integer string=w1914:string)  [unwired: 1 in]
                      n1479 = GPIB Write(0:w1914, 1:"OUTR?1") -> (6:w1920:errorcluster)  [unwired: 3 in, 1 out]
                      n1480 = GPIB Read(0:w1914, 1:3200, 3:w1920) -> (5:w1918:string)  [unwired: 2 in, 2 out]
                      n1481 = Fract/Exp String To Number(string=w1918) -> (number=w1917:dbl)  [unwired: 3 in, 1 out]
                      n1482 = Build Array (concatenate)(w1922, w1917) -> (w1921:dbl[])
                    }
                  }
                  n1483 = property on="data" class="Arr (strict)"("Value"=w1912) -> ()  [unwired: 2 in, 2 out]
                }
                frame #1 {
                  # "check if out-of-phase\nsignal on lock-in 1 \nis to be measured"
                  n1484 = property on="data" class="Arr (strict)"() -> ("Value"=w1924:dbl[])  [unwired: 2 in, 2 out]
                  n1485 = local read "SR830 1 oop"() -> (w1923:bool)
                  n1486 = case shown="True" w1923 {
                    tunnel: w1924 -> [w1926 w1935]
                    tunnel: [w1926 w1934] -> w1925
                    frame False {
                      # "we are not measuring out of phase signal on lock-in 1 (SR830_1_oop)"
                    }
                    frame True {
                      # "we are  measuring lock-in 1, out of phase (SR830_1_oop)"
                      n1487 = local read "SR830 1 addr"() -> (w1928:u8)
                      n1488 = Number To Decimal String(number=w1928) -> (decimal integer string=w1927:string)  [unwired: 1 in]
                      n1489 = GPIB Write(0:w1927, 1:"OUTR?2") -> (6:w1933:errorcluster)  [unwired: 3 in, 1 out]
                      n1490 = GPIB Read(0:w1927, 1:3200, 3:w1933) -> (5:w1931:string)  [unwired: 2 in, 2 out]
                      n1491 = Fract/Exp String To Number(string=w1931) -> (number=w1930:dbl)  [unwired: 3 in, 1 out]
                      n1492 = Build Array (concatenate)(w1935, w1930) -> (w1934:dbl[])
                    }
                  }
                  n1493 = property on="data" class="Arr (strict)"("Value"=w1925) -> ()  [unwired: 2 in, 2 out]
                }
                frame #2 {
                  # "check if in-phase\nsignal on lock-in 2 \nis to be measured"
                  n1494 = property on="data" class="Arr (strict)"() -> ("Value"=w1937:dbl[])  [unwired: 2 in, 2 out]
                  n1495 = local read "SR830 2 ip"() -> (w1936:bool)
                  n1496 = case shown="True" w1936 {
                    tunnel: w1937 -> [w1939 w1948]
                    tunnel: [w1939 w1947] -> w1938
                    frame False {
                      # "we are not measuring in phase signal on lock-in 2 (SR830_2_ip)"
                    }
                    frame True {
                      # "we are  measuring lock-in 2, in phase (SR830_2_ip)"
                      n1497 = local read "SR830 2 addr"() -> (w1941:u8)
                      n1498 = Number To Decimal String(number=w1941) -> (decimal integer string=w1940:string)  [unwired: 1 in]
                      n1499 = GPIB Write(0:w1940, 1:"OUTP?1") -> (6:w1946:errorcluster)  [unwired: 3 in, 1 out]
                      n1500 = GPIB Read(0:w1940, 1:3200, 3:w1946) -> (5:w1944:string)  [unwired: 2 in, 2 out]
                      n1501 = Fract/Exp String To Number(string=w1944) -> (number=w1943:dbl)  [unwired: 3 in, 1 out]
                      n1502 = Build Array (concatenate)(w1948, w1943) -> (w1947:dbl[])
                    }
                  }
                  n1503 = property on="data" class="Arr (strict)"("Value"=w1938) -> ()  [unwired: 2 in, 2 out]
                }
                frame #3 {
                  # "check if out-of-phase\nsignal on lock-in 2 \nis to be measured"
                  n1504 = property on="data" class="Arr (strict)"() -> ("Value"=w1950:dbl[])  [unwired: 2 in, 2 out]
                  n1505 = local read "SR830 2 oop"() -> (w1949:bool)
                  n1506 = case shown="True" w1949 {
                    tunnel: w1950 -> [w1952 w1961]
                    tunnel: [w1952 w1960] -> w1951
                    frame False {
                      # "we are not measuring out of phase signal on lock-in 2 (SR830_2_oop)"
                    }
                    frame True {
                      # "we are  measuring lock-in 2, out of phase (SR830_2_oop)"
                      n1507 = local read "SR830 2 addr"() -> (w1954:u8)
                      n1508 = Number To Decimal String(number=w1954) -> (decimal integer string=w1953:string)  [unwired: 1 in]
                      n1509 = GPIB Write(0:w1953, 1:"OUTP?2") -> (6:w1959:errorcluster)  [unwired: 3 in, 1 out]
                      n1510 = GPIB Read(0:w1953, 1:3200, 3:w1959) -> (5:w1957:string)  [unwired: 2 in, 2 out]
                      n1511 = Fract/Exp String To Number(string=w1957) -> (number=w1956:dbl)  [unwired: 3 in, 1 out]
                      n1512 = Build Array (concatenate)(w1961, w1956) -> (w1960:dbl[])
                    }
                  }
                  n1513 = property on="data" class="Arr (strict)"("Value"=w1951) -> ()  [unwired: 2 in, 2 out]
                }
                frame #4 {
                  # "check if in-phase\nsignal on lock-in 3 \nis to be measured"
                  n1514 = property on="data" class="Arr (strict)"() -> ("Value"=w1963:dbl[])  [unwired: 2 in, 2 out]
                  n1515 = local read "SR830 3 ip"() -> (w1962:bool)
                  n1516 = case shown="True" w1962 {
                    tunnel: w1963 -> [w1965 w1974]
                    tunnel: [w1965 w1973] -> w1964
                    frame False {
                      # "we are not measuring in phase signal on lock-in 3 (SR830_3_ip)"
                    }
                    frame True {
                      # "we are  measuring lock-in 3, in phase (SR830_3_ip)"
                      n1517 = local read "SR830 3 addr"() -> (w1967:u8)
                      n1518 = Number To Decimal String(number=w1967) -> (decimal integer string=w1966:string)  [unwired: 1 in]
                      n1519 = GPIB Write(0:w1966, 1:"OUTP?1") -> (6:w1972:errorcluster)  [unwired: 3 in, 1 out]
                      n1520 = GPIB Read(0:w1966, 1:3200, 3:w1972) -> (5:w1970:string)  [unwired: 2 in, 2 out]
                      n1521 = Fract/Exp String To Number(string=w1970) -> (number=w1969:dbl)  [unwired: 3 in, 1 out]
                      n1522 = Build Array (concatenate)(w1974, w1969) -> (w1973:dbl[])
                    }
                  }
                  n1523 = property on="data" class="Arr (strict)"("Value"=w1964) -> ()  [unwired: 2 in, 2 out]
                }
                frame #5 {
                  # "check if out-of-phase\nsignal on lock-in 3 \nis to be measured"
                  n1524 = property on="data" class="Arr (strict)"() -> ("Value"=w1976:dbl[])  [unwired: 2 in, 2 out]
                  n1525 = local read "SR830 3 oop"() -> (w1975:bool)
                  n1526 = case shown="True" w1975 {
                    tunnel: w1976 -> [w1978 w1987]
                    tunnel: [w1978 w1986] -> w1977
                    frame False {
                      # "we are not measuring out of phase signal on lock-in 3 (SR830_3_oop)"
                    }
                    frame True {
                      # "we are  measuring lock-in 3, out of phase (SR830_3_oop)"
                      n1527 = local read "SR830 3 addr"() -> (w1980:u8)
                      n1528 = Number To Decimal String(number=w1980) -> (decimal integer string=w1979:string)  [unwired: 1 in]
                      n1529 = GPIB Write(0:w1979, 1:"OUTP?2") -> (6:w1985:errorcluster)  [unwired: 3 in, 1 out]
                      n1530 = GPIB Read(0:w1979, 1:3200, 3:w1985) -> (5:w1983:string)  [unwired: 2 in, 2 out]
                      n1531 = Fract/Exp String To Number(string=w1983) -> (number=w1982:dbl)  [unwired: 3 in, 1 out]
                      n1532 = Build Array (concatenate)(w1987, w1982) -> (w1986:dbl[])
                    }
                  }
                  n1533 = property on="data" class="Arr (strict)"("Value"=w1977) -> ()  [unwired: 2 in, 2 out]
                }
                frame #6 {
                  # "check if in-phase\nsignal on lock-in 4 \nis to be measured"
                  n1534 = property on="data" class="Arr (strict)"() -> ("Value"=w1989:dbl[])  [unwired: 2 in, 2 out]
                  n1535 = local read "SR830 4 ip"() -> (w1988:bool)
                  n1536 = case shown="True" w1988 {
                    tunnel: w1989 -> [w1991 w2000]
                    tunnel: [w1991 w1999] -> w1990
                    frame False {
                      # "we are not measuring in phase signal on lock-in 4 (SR830_4_ip)"
                    }
                    frame True {
                      # "we are  measuring lock-in 4, in phase (SR830_4_ip)"
                      n1537 = local read "SR830 4 addr"() -> (w1993:u8)
                      n1538 = Number To Decimal String(number=w1993) -> (decimal integer string=w1992:string)  [unwired: 1 in]
                      n1539 = GPIB Write(0:w1992, 1:"OUTP?1") -> (6:w1998:errorcluster)  [unwired: 3 in, 1 out]
                      n1540 = GPIB Read(0:w1992, 1:3200, 3:w1998) -> (5:w1996:string)  [unwired: 2 in, 2 out]
                      n1541 = Fract/Exp String To Number(string=w1996) -> (number=w1995:dbl)  [unwired: 3 in, 1 out]
                      n1542 = Build Array (concatenate)(w2000, w1995) -> (w1999:dbl[])
                    }
                  }
                  n1543 = property on="data" class="Arr (strict)"("Value"=w1990) -> ()  [unwired: 2 in, 2 out]
                }
                frame #7 {
                  # "check if out-of-phase\nsignal on lock-in 4 \nis to be measured"
                  n1544 = property on="data" class="Arr (strict)"() -> ("Value"=w2002:dbl[])  [unwired: 2 in, 2 out]
                  n1545 = local read "SR830 4 oop"() -> (w2001:bool)
                  n1546 = case shown="True" w2001 {
                    tunnel: w2002 -> [w2004 w2013]
                    tunnel: [w2004 w2012] -> w2003
                    frame False {
                      # "we are not measuring out of phase signal on lock-in 4 (SR830_4_oop)"
                    }
                    frame True {
                      # "we are  measuring lock-in 4, out of phase (SR830_4_oop)"
                      n1547 = local read "SR830 4 addr"() -> (w2006:u8)
                      n1548 = Number To Decimal String(number=w2006) -> (decimal integer string=w2005:string)  [unwired: 1 in]
                      n1549 = GPIB Write(0:w2005, 1:"OUTP?2") -> (6:w2011:errorcluster)  [unwired: 3 in, 1 out]
                      n1550 = GPIB Read(0:w2005, 1:3200, 3:w2011) -> (5:w2009:string)  [unwired: 2 in, 2 out]
                      n1551 = Fract/Exp String To Number(string=w2009) -> (number=w2008:dbl)  [unwired: 3 in, 1 out]
                      n1552 = Build Array (concatenate)(w2013, w2008) -> (w2012:dbl[])
                    }
                  }
                  n1553 = property on="data" class="Arr (strict)"("Value"=w2003) -> ()  [unwired: 2 in, 2 out]
                }
                frame #8 {
                  # "check if voltage \non 2400 SouceMeter 1\nis to be measured"
                  n1554 = property on="data" class="Arr (strict)"() -> ("Value"=w2015:dbl[])  [unwired: 2 in, 2 out]
                  n1555 = local read "2400 1 meas v"() -> (w2014:bool)
                  n1556 = case shown="True" w2014 {
                    tunnel: w2015 -> [w2017 w2028]
                    tunnel: [w2017 w2027] -> w2016
                    frame False {
                      # "we are not measuring 2400 1, voltage (2400_1_v)"
                    }
                    frame True {
                      # "we are  measuring 2400 1, voltage (2400_1_v)"
                      n1557 = local read "2400 1 addr"() -> (w2022:u8)
                      n1558 = Number To Decimal String(number=w2022) -> (decimal integer string=w2021:string)  [unwired: 1 in]
                      n1559 = GPIB Write(0:w2021, 1:":READ?") -> (6:w2026:errorcluster)  [unwired: 3 in, 1 out]
                      n1560 = GPIB Read(0:w2021, 1:3200, 3:w2026) -> (5:w2019:string)  [unwired: 2 in, 2 out]
                      n1561 = String Subset(string=w2019, length (rest)=13) -> (substring=w2018:string)  [unwired: 1 in]
                      n1562 = Fract/Exp String To Number(string=w2018) -> (number=w2024:dbl)  [unwired: 3 in, 1 out]
                      n1563 = Build Array (concatenate)(w2028, w2024) -> (w2027:dbl[])
                    }
                  }
                  n1564 = property on="data" class="Arr (strict)"("Value"=w2016) -> ()  [unwired: 2 in, 2 out]
                }
                frame #9 {
                  # "check if current \non 2400 SouceMeter 1\nis to be measured"
                  n1565 = property on="data" class="Arr (strict)"() -> ("Value"=w2030:dbl[])  [unwired: 2 in, 2 out]
                  n1566 = local read "2400 1 meas i"() -> (w2029:bool)
                  n1567 = case shown="True" w2029 {
                    tunnel: w2030 -> [w2032 w2044]
                    tunnel: [w2032 w2043] -> w2031
                    frame False {
                      # "we are not measuring 2400 1, current (2400_1_i)"
                    }
                    frame True {
                      # "we are  measuring 2400 1, current (2400_1_i)"
                      n1568 = local read "2400 1 addr"() -> (w2038:u8)
                      n1569 = Number To Decimal String(number=w2038) -> (decimal integer string=w2037:string)  [unwired: 1 in]
                      n1570 = GPIB Write(0:w2037, 1:":READ?") -> (6:w2042:errorcluster)  [unwired: 3 in, 1 out]
                      n1571 = GPIB Read(0:w2037, 1:3200, 3:w2042) -> (5:w2035:string)  [unwired: 2 in, 2 out]
                      n1572 = String Subset(string=w2035, offset (0)=14, length (rest)=13) -> (substring=w2034:string)
                      n1573 = Fract/Exp String To Number(string=w2034) -> (number=w2040:dbl)  [unwired: 3 in, 1 out]
                      n1574 = Build Array (concatenate)(w2044, w2040) -> (w2043:dbl[])
                    }
                  }
                  n1575 = property on="data" class="Arr (strict)"("Value"=w2031) -> ()  [unwired: 2 in, 2 out]
                }
                frame #10 {
                  # "check if voltage \non 2400 SouceMeter 2\nis to be measured"
                  n1576 = property on="data" class="Arr (strict)"() -> ("Value"=w2046:dbl[])  [unwired: 2 in, 2 out]
                  n1577 = local read "2400 2 meas v"() -> (w2045:bool)
                  n1578 = case shown="True" w2045 {
                    tunnel: w2046 -> [w2048 w2059]
                    tunnel: [w2048 w2058] -> w2047
                    frame False {
                      # "we are not measuring 2400 2, voltage (2400_2_v)"
                    }
                    frame True {
                      # "we are  measuring 2400 2, voltage (2400_2_v)"
                      n1579 = local read "2400 2 addr"() -> (w2053:u8)
                      n1580 = Number To Decimal String(number=w2053) -> (decimal integer string=w2052:string)  [unwired: 1 in]
                      n1581 = GPIB Write(0:w2052, 1:":READ?") -> (6:w2057:errorcluster)  [unwired: 3 in, 1 out]
                      n1582 = GPIB Read(0:w2052, 1:3200, 3:w2057) -> (5:w2050:string)  [unwired: 2 in, 2 out]
                      n1583 = String Subset(string=w2050, length (rest)=13) -> (substring=w2049:string)  [unwired: 1 in]
                      n1584 = Fract/Exp String To Number(string=w2049) -> (number=w2055:dbl)  [unwired: 3 in, 1 out]
                      n1585 = Build Array (concatenate)(w2059, w2055) -> (w2058:dbl[])
                    }
                  }
                  n1586 = property on="data" class="Arr (strict)"("Value"=w2047) -> ()  [unwired: 2 in, 2 out]
                }
                frame #11 {
                  # "check if current \non 2400 SouceMeter 2\nis to be measured"
                  n1587 = property on="data" class="Arr (strict)"() -> ("Value"=w2061:dbl[])  [unwired: 2 in, 2 out]
                  n1588 = local read "2400 2 meas i"() -> (w2060:bool)
                  n1589 = case shown="True" w2060 {
                    tunnel: w2061 -> [w2063 w2075]
                    tunnel: [w2063 w2074] -> w2062
                    frame False {
                      # "we are not measuring 2400 2, current (2400_2_i)"
                    }
                    frame True {
                      # "we are  measuring 2400 2, current (2400_2_i)"
                      n1590 = local read "2400 2 addr"() -> (w2069:u8)
                      n1591 = Number To Decimal String(number=w2069) -> (decimal integer string=w2068:string)  [unwired: 1 in]
                      n1592 = GPIB Write(0:w2068, 1:":READ?") -> (6:w2073:errorcluster)  [unwired: 3 in, 1 out]
                      n1593 = GPIB Read(0:w2068, 1:3200, 3:w2073) -> (5:w2066:string)  [unwired: 2 in, 2 out]
                      n1594 = String Subset(string=w2066, offset (0)=14, length (rest)=13) -> (substring=w2065:string)
                      n1595 = Fract/Exp String To Number(string=w2065) -> (number=w2071:dbl)  [unwired: 3 in, 1 out]
                      n1596 = Build Array (concatenate)(w2075, w2071) -> (w2074:dbl[])
                    }
                  }
                  n1597 = property on="data" class="Arr (strict)"("Value"=w2062) -> ()  [unwired: 2 in, 2 out]
                }
                frame #12 {
                  # "check if voltage \non 2400 SouceMeter 3\nis to be measured"
                  n1598 = property on="data" class="Arr (strict)"() -> ("Value"=w2077:dbl[])  [unwired: 2 in, 2 out]
                  n1599 = local read "2400 3 meas v"() -> (w2076:bool)
                  n1600 = case shown="True" w2076 {
                    tunnel: w2077 -> [w2079 w2090]
                    tunnel: [w2079 w2089] -> w2078
                    frame False {
                      # "we are not measuring 2400 3, voltage (2400_3_v)"
                    }
                    frame True {
                      # "we are  measuring 2400 3, voltage (2400_3_v)"
                      n1601 = local read "2400 3 addr"() -> (w2084:u8)
                      n1602 = Number To Decimal String(number=w2084) -> (decimal integer string=w2083:string)  [unwired: 1 in]
                      n1603 = GPIB Write(0:w2083, 1:":READ?") -> (6:w2088:errorcluster)  [unwired: 3 in, 1 out]
                      n1604 = GPIB Read(0:w2083, 1:3200, 3:w2088) -> (5:w2081:string)  [unwired: 2 in, 2 out]
                      n1605 = String Subset(string=w2081, length (rest)=13) -> (substring=w2080:string)  [unwired: 1 in]
                      n1606 = Fract/Exp String To Number(string=w2080) -> (number=w2086:dbl)  [unwired: 3 in, 1 out]
                      n1607 = Build Array (concatenate)(w2090, w2086) -> (w2089:dbl[])
                    }
                  }
                  n1608 = property on="data" class="Arr (strict)"("Value"=w2078) -> ()  [unwired: 2 in, 2 out]
                }
                frame #13 {
                  # "check if current \non 2400 SouceMeter 3\nis to be measured"
                  n1609 = property on="data" class="Arr (strict)"() -> ("Value"=w2092:dbl[])  [unwired: 2 in, 2 out]
                  n1610 = local read "2400 3 meas i"() -> (w2091:bool)
                  n1611 = case shown="True" w2091 {
                    tunnel: w2092 -> [w2094 w2106]
                    tunnel: [w2094 w2105] -> w2093
                    frame False {
                      # "we are not measuring 2400 3, current (2400_3_i)"
                    }
                    frame True {
                      # "we are  measuring 2400 3, current (2400_3_i)"
                      n1612 = local read "2400 3 addr"() -> (w2100:u8)
                      n1613 = Number To Decimal String(number=w2100) -> (decimal integer string=w2099:string)  [unwired: 1 in]
                      n1614 = GPIB Write(0:w2099, 1:":READ?") -> (6:w2104:errorcluster)  [unwired: 3 in, 1 out]
                      n1615 = GPIB Read(0:w2099, 1:3200, 3:w2104) -> (5:w2097:string)  [unwired: 2 in, 2 out]
                      n1616 = String Subset(string=w2097, offset (0)=14, length (rest)=13) -> (substring=w2096:string)
                      n1617 = Fract/Exp String To Number(string=w2096) -> (number=w2102:dbl)  [unwired: 3 in, 1 out]
                      n1618 = Build Array (concatenate)(w2106, w2102) -> (w2105:dbl[])
                    }
                  }
                  n1619 = property on="data" class="Arr (strict)"("Value"=w2093) -> ()  [unwired: 2 in, 2 out]
                }
                frame #14 {
                  # "check if 1st channel \non Keithley 2182A 1\nis to be measured"
                  n1620 = property on="data" class="Arr (strict)"() -> ("Value"=w2108:dbl[])  [unwired: 2 in, 2 out]
                  n1621 = local read "2182A 1 ch1"() -> (w2107:bool)
                  n1622 = case shown="True" w2107 {
                    tunnel: w2108 -> [w2110 w2119]
                    tunnel: [w2110 w2118] -> w2109
                    frame False {
                      # "we are not measuring 2182A 1 channel 1 (2182A_1_ch1)"
                    }
                    frame True {
                      # "we are  measuring 2182A 1 channel 1 (2182A_1_ch1)"
                      n1623 = local read "2182A 1 addr"() -> (w2113:u8)
                      n1624 = Number To Decimal String(number=w2113) -> (decimal integer string=w2112:string)  [unwired: 1 in]
                      n1625 = GPIB Write(0:w2112, 1:":SENSe:DATA:FRES?") -> (6:w2117:errorcluster)  [unwired: 3 in, 1 out]
                      n1626 = GPIB Read(0:w2112, 1:200, 3:w2117) -> (5:w2111:string)  [unwired: 2 in, 2 out]
                      n1627 = Fract/Exp String To Number(string=w2111) -> (number=w2115:dbl)  [unwired: 3 in, 1 out]
                      n1628 = Build Array (concatenate)(w2119, w2115) -> (w2118:dbl[])
                    }
                  }
                  n1629 = property on="data" class="Arr (strict)"("Value"=w2109) -> ()  [unwired: 2 in, 2 out]
                }
                frame #15 {
                  # "check if 2nd channel \non Keithley 2182A 1\nis to be measured"
                  n1630 = property on="data" class="Arr (strict)"() -> ("Value"=w2121:dbl[])  [unwired: 2 in, 2 out]
                  n1631 = local read "2182A 1 ch2"() -> (w2120:bool)
                  n1632 = case shown="True" w2120 {
                    tunnel: w2121 -> [w2123 w2136]
                    tunnel: [w2123 w2135] -> w2122
                    frame False {
                      # "we are not measuring 2182A 1 channel 2 (2182A_1_ch2)"
                    }
                    frame True {
                      # "switching to channel 2 and then\nback to channel 1"
                      # "we are  measuring 2182A 1 channel 2 (2182A_1_ch2)"
                      n1633 = local read "2182A 1 addr"() -> (w2130:u8)
                      n1634 = Number To Decimal String(number=w2130) -> (decimal integer string=w2125:string)  [unwired: 1 in]
                      n1635 = GPIB Write(0:w2125, 1:":SENSe:CHAN 2") -> (6:w2127:errorcluster)  [unwired: 3 in, 1 out]
                      n1636 = GPIB Write(0:w2125, 1:":SENSe:DATA:FRES?", 3:w2127) -> (6:w2134:errorcluster)  [unwired: 2 in, 1 out]
                      n1637 = GPIB Read(0:w2125, 1:200, 3:w2134) -> (5:w2129:string, 7:w2126:errorcluster)  [unwired: 2 in, 1 out]
                      n1638 = GPIB Write(0:w2125, 1:":SENSe:CHAN 1", 3:w2126) -> ()  [unwired: 2 in, 2 out]
                      n1639 = Fract/Exp String To Number(string=w2129) -> (number=w2132:dbl)  [unwired: 3 in, 1 out]
                      n1640 = Build Array (concatenate)(w2136, w2132) -> (w2135:dbl[])
                    }
                  }
                  n1641 = property on="data" class="Arr (strict)"("Value"=w2122) -> ()  [unwired: 2 in, 2 out]
                }
                frame #16 {
                  # "check if 1st channel \non Keithley 2182A 2\nis to be measured"
                  n1642 = property on="data" class="Arr (strict)"() -> ("Value"=w2138:dbl[])  [unwired: 2 in, 2 out]
                  n1643 = local read "2182A 2 ch1"() -> (w2137:bool)
                  n1644 = case shown="True" w2137 {
                    tunnel: w2138 -> [w2140 w2149]
                    tunnel: [w2140 w2148] -> w2139
                    frame False {
                      # "we are not measuring 2182A 2 channel 1 (2182A_2_ch1)"
                    }
                    frame True {
                      # "we are  measuring 2182A 2 channel 1 (2182A_2_ch1)"
                      n1645 = local read "2182A 2 addr"() -> (w2143:u8)
